vi "create.DeleteOrder.vi"(8 "error in (no error)":errorcluster, 11 "DeleteOrder.Parameters":T1={"Time Offset"=447000, "Order Id"="ORID0001"}) -> (0 "error out":errorcluster, 2 "Bytes.out":u8[](array[numeric]) format="%.0x", 3 "MessageBase out":refnum<class "DeleteOrder.lvclass">)   [LabVIEW 2022 SP3]
uses:
  DeleteOrder/DeleteOrder.Parameters.ctl
  DeleteOrder/DeleteOrder.lvclass
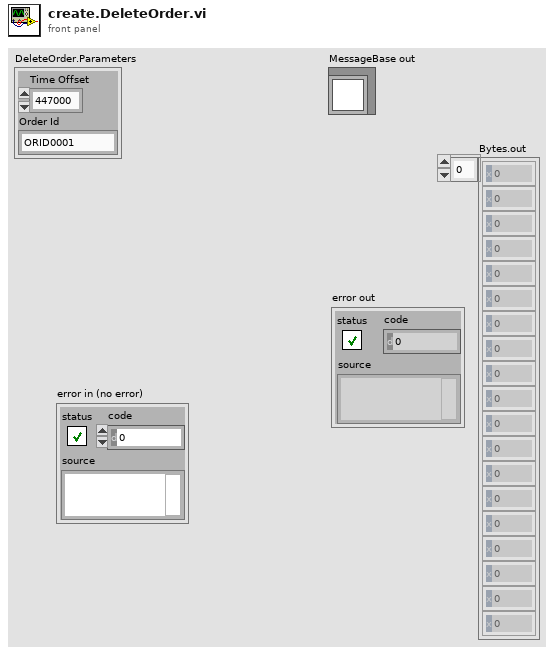
[diagram p1: front panel]
types:
  T1 = typedef "DeleteOrder.lvclass/DeleteOrder.Parameters.ctl" = cluster{"Time Offset":u32, "Order Id":string}
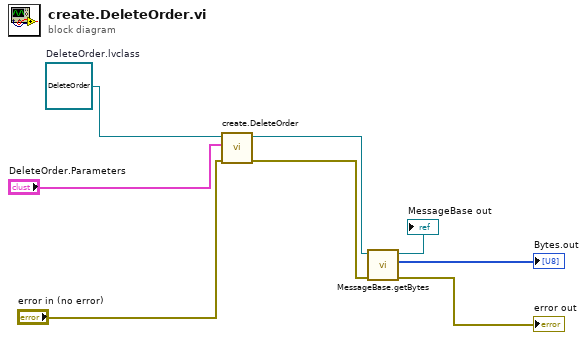
[diagram p0: block diagram]
diagram:
  w6 = refnum<class "DeleteOrder.lvclass"> refnum  # DeleteOrder.lvclass
  n1 = call-dynamic "create.DeleteOrder.vi"("error in"="error in (no error)", "DeleteOrder.Parameters"="DeleteOrder.Parameters", "DeleteOrder in"=w6) -> ("error out"=w3:errorcluster, "DeleteOrder out"=w2:refnum<class "DeleteOrder.lvclass">)  [unwired: 7 in]
  n2 = call-dynamic "MessageBase.getBytes.vi"("error in (no error)"=w3, "MessageBase in"=w2) -> ("error out"=→"error out":errorcluster, "Bytes.out"=→"Bytes.out":u8[], "MessageBase out"=→"MessageBase out":refnum<class "DeleteOrder.lvclass">)  [unwired: 7 in]
